vi "Calculate Fit.vi"(9 "Response in":dbl[][](array[numeric]), 10 "Stimulus in":dbl[][](array[numeric]), 11 "Exponential Fit in":refnum<class "Exponential Fit.lvclass">) -> (3 "Exponential Fit out":refnum<class "Exponential Fit.lvclass">)   [LabVIEW 2013, in "Exponential Fit.lvclass"]
uses:
  Exponential Fit.lvclass
  <vilib>/Analysis/6fits.llb/Curve Fitting Criteria.ctl
  Exponential Fit.lvclass/Exponential Fit.ctl
  <vilib>/Analysis/NI_AALPro.lvlib
  Abstract Fit/Abstract Fit.lvclass
  comm/nan operations/nan operations.lvlib
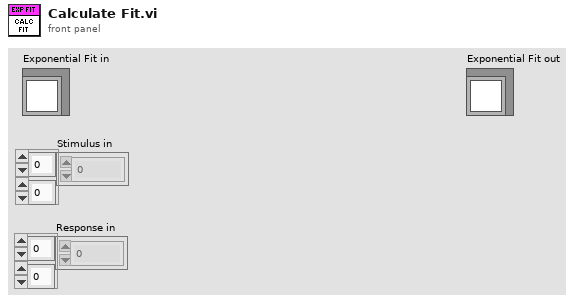
[diagram p1: front panel]
types:
  T1 = cluster{"amp min":dbl, "amp max":dbl, "damping min":dbl, "damping max":dbl, "offset min":dbl, "offset max":dbl}
  T2 = typedef "NI_AALPro.lvlib/Curve Fitting Criteria.ctl" = u16
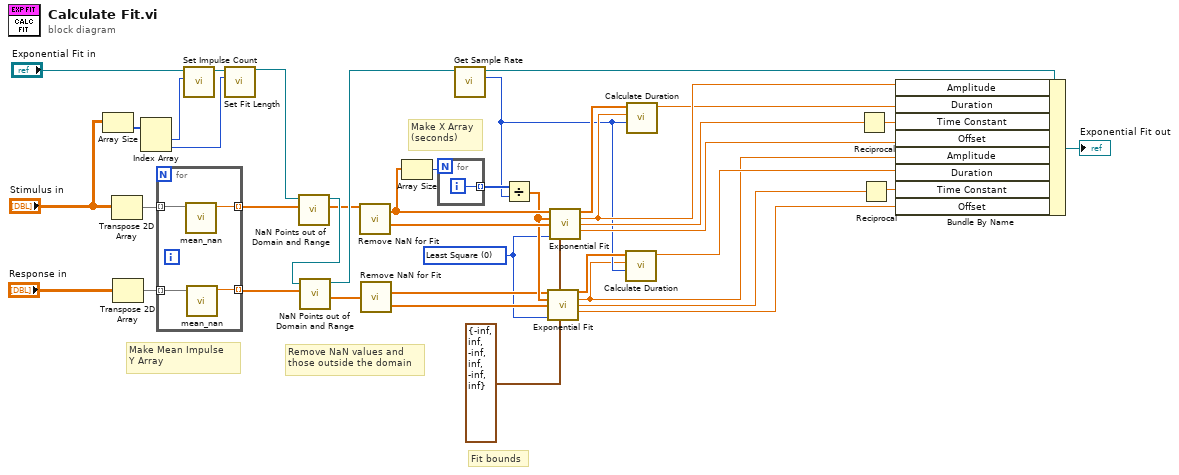
[diagram p0: block diagram]
diagram:
  w8 = T1 {"amp min"=-inf, "amp max"=inf, "damping min"=-inf, "damping max"=inf, "offset min"=-inf, "offset max"=inf} ("parameter bounds")
  w16 = T2 0 items=["Least Square", "Least Absolute Residual", "Bisquare"] ("method")
  # "Fit bounds"
  # "Remove NaN values and \nthose outside the domain"
  # "Make Mean Impulse \nY Array"
  # "Make X Array\n(seconds)"
  n1 = Array Size(array="Stimulus in") -> (size(s)=w36:i32[])
  n2 = Transpose 2D Array(2D array="Stimulus in") -> (transposed array=w32:dbl[][])
  n3 = Transpose 2D Array(2D array="Response in") -> (transposed array=w33:dbl[][])
  n4 = Index Array(array=w36) -> (element #1=w37:i32, element #2=w39:i32)  [unwired: 2 in]
  n5 = for {
    tunnel: w32 -> [w44] mode=indexing
    tunnel: w33 -> [w43] mode=indexing
    tunnel: [w42] -> w3 mode=indexing
    tunnel: [w41] -> w2 mode=indexing
    n6 = call "mean_nan.vi"("Array"=w44) -> ("Mean"=w42:dbl)  [unwired: 10 in]
    n7 = call "mean_nan.vi"("Array"=w43) -> ("Mean"=w41:dbl)  [unwired: 10 in]
  }
  n8 = call-dynamic "Set Impulse Count.vi"("Nr of Fit Impulses"=w37, "Abstract Fit in"="Exponential Fit in") -> ("Abstract Fit out"=w38:refnum<class "Exponential Fit.lvclass">)  [unwired: 8 in, 1 out]
  n9 = call-dynamic "Set Fit Length.vi"("Length"=w39, "Abstract Fit in"=w38) -> ("Abstract Fit out"=w5:refnum<class "Exponential Fit.lvclass">)  [unwired: 8 in, 1 out]
  n10 = call "NaN Points out of Domain and Range.vi"("Data in"=w3, "Exponential Fit in"=w5) -> ("Data out"=w4:dbl[], "Exponential Fit out"=w7:refnum<class "Exponential Fit.lvclass">)  [unwired: 8 in]
  n11 = call "NaN Points out of Domain and Range.vi"("Data in"=w2, "Exponential Fit in"=w7) -> ("Data out"=w1:dbl[], "Exponential Fit out"=w6:refnum<class "Exponential Fit.lvclass">)  [unwired: 8 in]
  n12 = call "Remove NaN for Fit.vi"("Data in"=w4) -> ("Weight out"=w29:dbl[], "Data out"=w28:dbl[])  [unwired: 2 in]
  n13 = call "Remove NaN for Fit.vi"("Data in"=w1) -> ("Weight out"=w17:dbl[], "Data out"=w18:dbl[])  [unwired: 2 in]
  n14 = Array Size(array=w28) -> (size(s)=w27:i32)
  n15 = for {
    N: w27 -> [_]
    tunnel: [w45] -> w26 mode=indexing
    i -> [w45]
  }
  n16 = call-dynamic "Get Sample Rate.vi"("Abstract Fit in"=w6) -> ("Sample Rate"=w14:i32, "Abstract Fit out"=w34:refnum<class "Exponential Fit.lvclass">)  [unwired: 8 in, 1 out]
  n17 = Divide(x=w26, y=w14) -> (x/y=w19:dbl[])
  n18 = call <vilib>:"Exponential Fit.vi"("Y"=w18, "X"=w19, "Weight"=w17, "method"=w16, "parameter bounds"=w8) -> ("Best Exponential Fit"=w15:dbl[], "amplitude"=w9:dbl, "damping"=w12:dbl, "offset"=w11:dbl)  [unwired: 5 in, 2 out]
  n19 = call <vilib>:"Exponential Fit.vi"("Y"=w28, "X"=w19, "Weight"=w29, "method"=w16, "parameter bounds"=w8) -> ("Best Exponential Fit"=w22:dbl[], "amplitude"=w21:dbl, "damping"=w24:dbl, "offset"=w25:dbl)  [unwired: 5 in, 2 out]
  n20 = call "Calculate Duration.vi"("Sample Rate"=w14, "Amplitude"=w9, "Y Values"=w15) -> ("Duration"=w10:dbl)  [unwired: 8 in]
  n21 = call "Calculate Duration.vi"("Sample Rate"=w14, "Amplitude"=w21, "Y Values"=w22) -> ("Duration"=w20:dbl)  [unwired: 8 in]
  n22 = Reciprocal(x=w24) -> (1/x=w23:dbl)
  n23 = Reciprocal(x=w12) -> (1/x=w13:dbl)
  n24 = Bundle By Name(cluster=w34, "Amplitude"=w21, "Duration"=w20, "Time Constant"=w23, "Offset"=w25, "Amplitude"=w9, "Duration"=w10, "Time Constant"=w13, "Offset"=w11) -> (→"Exponential Fit out":refnum<class "Exponential Fit.lvclass">)
